vi "EMG_Control.vi"() -> ()   [LabVIEW 2015]
uses:
  <instrlib>/Dynamixel Motor/Public/Motor Operation/Low Level/Baud Setting.ctl
  <vilib>/Platform/TimedLoop/XDataNode/timing_clust.ctl
  <vilib>/Platform/TimedLoop/XDataNode/nitl_modes.ctl
  <vilib>/Platform/TimedLoop/XDataNode/wakeup.ctl
  <vilib>/platform/TimedLoop/XDataNode/XDataNode.xnode
  <instrlib>/Dynamixel Motor/Dynamixel Motor.lvlib
  <vilib>/Platform/TimedLoop/XDataNode/XDNodeRunTimeDep.lvlib
panel:
  out "Mover 4 motor info (degree)":T1(array[cluster]) {"Error Code (bits)" format="%b"}
  out "Hand motors info":T2(array[cluster])
  in  "Triceps max amplitude (V)":dbl
  in  "Biceps max amplitude (V)":dbl
  out "Mode":enum16{" M3", " M2", " M1"}(ring)
  in  "Positions":T3
  in  "Target IP Address":string="172.22.11.2"
  in  "VISA resource name":refnum<visa-resource-name>="COM9"
  in  "stop":bool
  out "Biceps EMG signal (V)":dbl[](graph)
  in  "Calibrate?":bool
  out "Biceps first threshold (V)":dbl
  out "Biceps second threshold (V)":dbl
  out "Triceps first threshold (V)":dbl
  out "Triceps second threshold (V)":dbl
  out "Triceps EMG signal (V)":dbl[](graph)
  out "Triceps hardly contracted?":bool
  out "Triceps contracted?":bool
  out "Biceps hardly contracted?":bool
  out "Biceps contracted?":bool
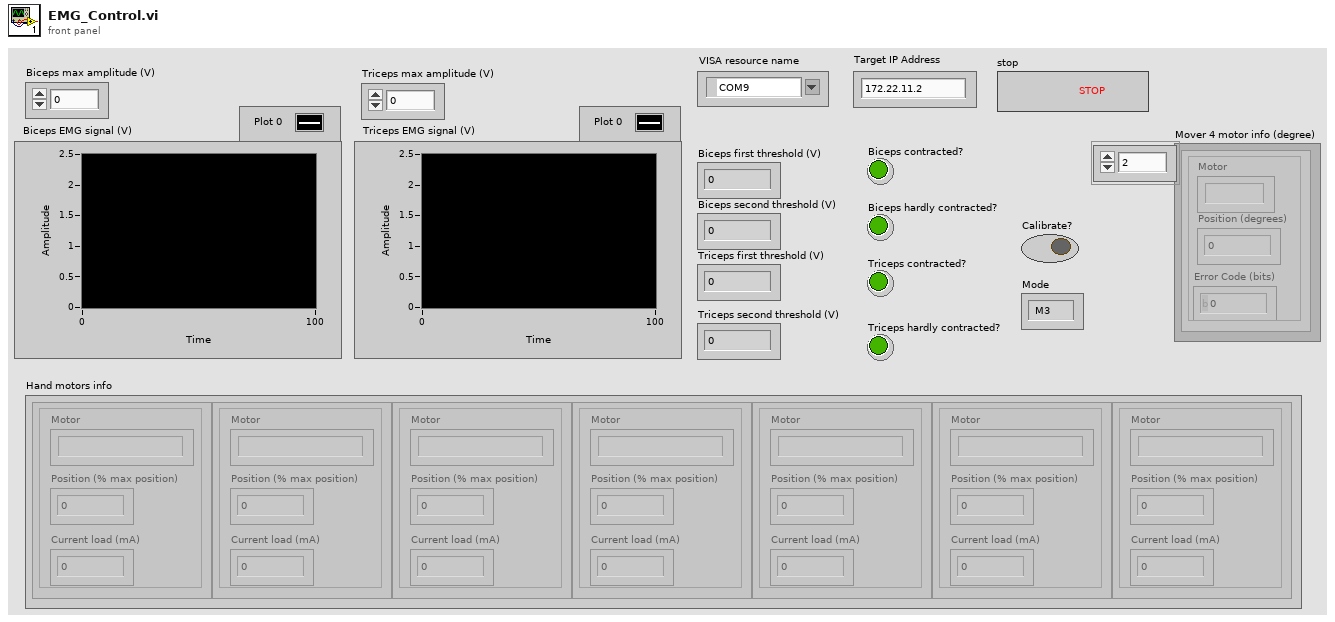
[diagram p1: front panel]
types:
  T1 = cluster{"Position (degrees)":i32, "Error Code (bits)":u8, "Motor":string}[]
  T2 = cluster{"Motor ":string, "Position (% max position)":dbl, "Current load (mA)":dbl}[]
  T3 = cluster{"ID":u16, "Position (bit)":u16, "Current load (mA)":u16}
  T4 = cluster{"Enable?":bool, "Reset?":bool, "EMG control":enum16{"Rest", "Biceps contracted", "Triceps contracted"}, "Motor speed":u8}
  T5 = cluster{"ID":u16, "Position (bit)":u16, "Current load (mA)":u16}[]
  T6 = cluster{"Read Access":enum8{"Allowed", "Required", "None"}, "Write Access":enum8{"Allowed", "Required", "None"}}
  T7 = cluster{"ID":u8, "Position":u16, "Error Code":u8}[]
  T8 = typedef "Dynamixel Motor.lvlib/Baud Setting.ctl" = u8
  T9 = typedef "XDNodeRunTimeDep.lvlib/timing_clust.ctl" = cluster{"Expected End [f-1]":u64, "Actual End [f-1]":u64, "Finished Late? [f-1]":bool, "Expected End [i-1]":u64, "Actual End [i-1]":u64, "Finished Late? [i-1]":bool, "Expected Start [i]":u64, "Actual Start [i]":u64, "Expected Start [f]":u64, "Actual Start [f]":u64, "Source Name":string, "Structure Name":string, "Period":i64, "Deadline":i64, "Offset":i64, "Start":i64, "Priority":i32, "Timeout":i32, "Mode":T10, "Wakeup Reason":T11, "Error":errorcluster, "Source Type":string, "Secondary Source Type":string, "Global End Time":u64, "Global Start Time":u64, "Frame Duration":u64, "Iteration Duration":u64, "Assigned CPU":i32, "I/O Scan Engine Mode":u32}
  T10 = typedef "XDNodeRunTimeDep.lvlib/nitl_modes.ctl" = enum32{"No Change", "Process missed periods, maintain original phase", "Discard missed periods, maintain original phase", "Process missed periods, ignore original phase", "Discard missed periods, ignore original phase"}
  T11 = typedef "XDNodeRunTimeDep.lvlib/wakeup.ctl" = enum32{"Normal", "Aborted", "Asynchronous wakeup", "Timing source error", "Timed loop error", "Timeout"}
  T12 = enum16{"Rest", "Triceps hardly contracted", "Triceps contracted", "Biceps hardly contracted", "Biceps contracted", "Change mode"}
  T13 = cluster{"Motor ":string, "Position (% Max position)":dbl, "Current load (mA)":dbl}[]
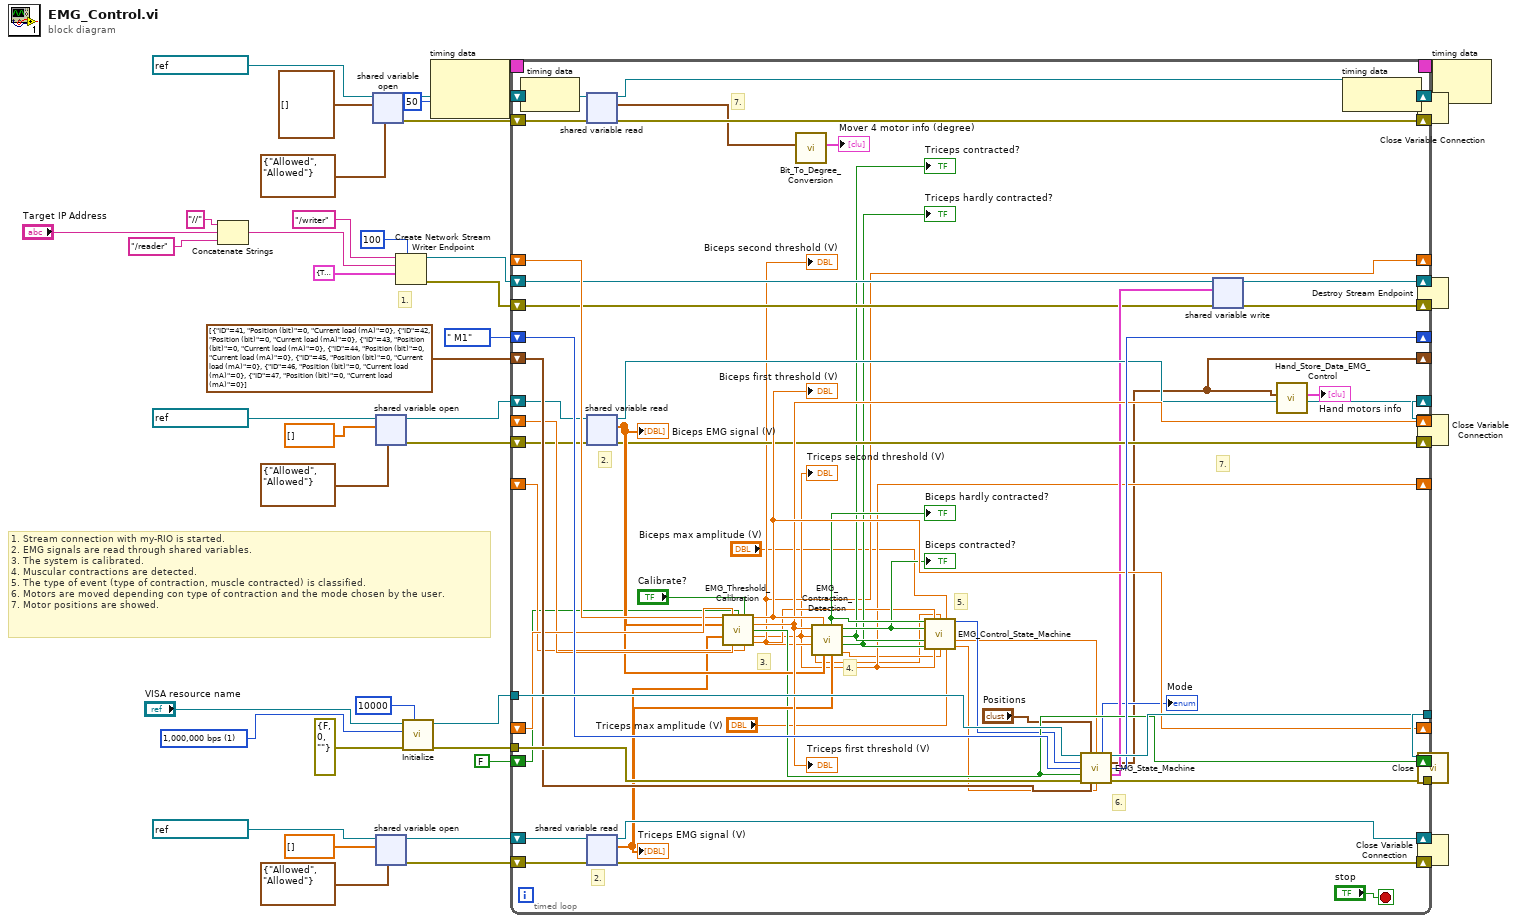
[diagram p0: block diagram]
diagram:
  w46 = T8 1 items=["1,000,000 bps"=1, "500,000 bps"=3, "400,000 bps"=4, "250,000 bps"=7, "200,000 bps"=9, "115200 bps"=16, "57600 bps"=34, "19200 bps"=103, "9600 bps"=207] ("Baud rate (57600 bps)")
  # "1."
  # "1. Stream connection with my-RIO is started.\n2. EMG signals are read through shared variables.\n3. The system is calibrated.\n4. Muscular contractions are detected.\n5. The type of event (type of contraction, muscle contracted) is classified.\n6. Motors are moved depending con type of contraction and the mode chosen by the user.\n7. Motor positions are showed."
  n1 = Concatenate Strings("//", "Target IP Address", "/reader") -> (w39:string)
  n2 = shared-variable-open(refnum<k21> "ni.var.psp://stratom-myrio/Shared_Variables/New position" ("shared variable refnum in"), T7 [] ("New position 2"), T6 {"Read Access"=enum."Allowed", "Write Access"=enum."Allowed"} ("access")) -> (w26:refnum<k21>, w24:errorcluster)  [unwired: 1 in]
  n3 = shared-variable-open(refnum<k21> "ni.var.psp://stratom-myrio/Shared_Variables/Biceps EMG signal" ("shared variable refnum in"), dbl[] [], T6 {"Read Access"=enum."Allowed", "Write Access"=enum."Allowed"} ("access")) -> (w18:refnum<k21>, w17:errorcluster)  [unwired: 1 in]
  n4 = shared-variable-open(refnum<k21> "ni.var.psp://stratom-myrio/Shared_Variables/Triceps EMG signal" ("shared variable refnum in"), dbl[] [], T6 {"Read Access"=enum."Allowed", "Write Access"=enum."Allowed"} ("access")) -> (w12:refnum<k21>, w11:errorcluster)  [unwired: 1 in]
  n5 = Create Network Stream Writer Endpoint(7:100 ("writer buffer size"), 9:T4 {"Enable?"=TRUE, "Reset?"=FALSE, "EMG control"=enum."Rest", "Motor speed"=0} ("data in"), 10:w39, 11:"/writer" ("reader name")) -> (0:w33:errorcluster, 3:w34:refnum<k21>)  [unwired: 3 in]
  n6 = call <instrlib>:"Initialize.vi"("Timeout (30 msec)"=u32 10000, "error in (no error)"=errorcluster {"status"=FALSE, "code"=0, "source"=""}, "Baud rate (57600 bps)"=w46, "VISA resource name"="VISA resource name") -> ("error out"=w41:errorcluster, "VISA resource name out"=w42:refnum<visa-resource-name>)  [unwired: 6 in]
  n7 = node-c288(i64 50 ("Period")) -> (w3:T9)  [unwired: 1 in]
  n8 = timed-loop {
    shift-right: [w85] -> _
    shift-left: _ -> [w89]
    shift-right: [w58] -> _
    shift-left: _ -> [w87]
    shift-right: [w84] -> _
    shift-left: _ -> [w88]
    shift-right: [w57] -> _
    shift-left: _ -> [w86]
    tunnel: w42 -> [w100]
    tunnel: w41 -> [w99]
    shift-right: [w66] -> w32
    shift-left: w34 -> [w67]
    shift-right: [w65] -> w31
    shift-left: w33 -> [w64]
    tunnel: [w97] -> w30
    tunnel: [w96] -> w29
    shift-right: [w95] -> _
    shift-left: enum16{" M3", " M2", " M1"}." M1" ("Mode Out") -> [w98]
    shift-right: [w50] -> _
    shift-left: T5 [{"ID"=41, "Position (bit)"=0, "Current load (mA)"=0}, {"ID"=42, "Position (bit)"=0, "Current load (mA)"=0}, {"ID"=43, "Position (bit)"=0, "Current load (mA)"=0}, {"ID"=44, "Position (bit)"=0, "Current load (mA)"=0}, {"ID"=45, "Position (bit)"=0, "Current load (mA)"=0}, {"ID"=46, "Position (bit)"=0, "Current load (mA)"=0}, {"ID"=47, "Position (bit)"=0, "Current load (mA)"=0}] ("New Hand Positions") -> [w94]
    shift-right: [w91] -> w23
    shift-left: w26 -> [w93]
    shift-right: [w90] -> w22
    shift-left: w24 -> [w92]
    shift-right: [w79] -> w10
    shift-left: w18 -> [w82]
    shift-right: [w78] -> w9
    shift-left: w17 -> [w81]
    shift-right: [w75] -> w8
    shift-left: w12 -> [w77]
    shift-right: [w74] -> w7
    shift-left: w11 -> [w76]
    shift-right: [w72] -> _
    shift-left: FALSE ("System calibrated?") -> [w71]
    timing: w3 -> [_]
    timing-out: [_] -> w2
    stop <- "stop" stop-if-true
    # "7."
    # "7."
    # "6."
    # "5."
    # "4."
    # "3."
    # "2."
    # "2."
    n9 = node-c288() -> ()  [unwired: 1 in, 1 out]
    n10 = shared-variable-read(w93, w92) -> (w91:refnum<k21>, w90:errorcluster, w48:T7)  [unwired: 1 out]
    n11 = shared-variable-read(w82, w81) -> (w79:refnum<k21>, w78:errorcluster, w80:dbl[])  [unwired: 1 out]
    "Biceps EMG signal (V)" <- w80
    n12 = shared-variable-read(w77, w76) -> (w75:refnum<k21>, w74:errorcluster, w73:dbl[])  [unwired: 1 out]
    "Triceps EMG signal (V)" <- w73
    n13 = call "EMG_Threshold_Calibration.vi"("Biceps harder contraction threshold in (V)"=w87, "Biceps contraction threshold in (V)"=w89, "System calibrated? (input)"=w71, "Calibrate?"="Calibrate?", "Biceps EMG signal (V)"=w80, "Triceps EMG signal (V)"=w73, "Triceps contraction threshold in (V)"=w88, "Triceps harderd contraction threshold in (V)"=w86) -> ("Biceps contraction threshold out (V)"=w85:dbl, "Triceps contraction threshold out (V)"=w84:dbl, "System calibrated?"=w72:bool, "Triceps harderd contraction threshold out (V)"=w57:dbl, "Biceps harder contraction threshold out (V)"=w58:dbl)  [unwired: 3 in]
    "Biceps first threshold (V)" <- w85
    "Biceps second threshold (V)" <- w58
    "Triceps first threshold (V)" <- w84
    "Triceps second threshold (V)" <- w57
    n14 = call "Bit_To_Degree_Conversion.vi"("Actual joints positions"=w48) -> ("Motor positions (degree)"=→"Mover 4 motor info (degree)":T1)  [unwired: 10 in]
    n15 = call "EMG_Contraction_Detection.vi"("Triceps EMG signal (V)"=w73, "Biceps EMG signal (V)"=w80, "Biceps contraction threshold (V)"=w85, "Biceps harder contraction threshold  (V)"=w58, "Triceps harderd contraction threshold  (V)"=w57, "Triceps contraction threshold  (V)"=w84) -> ("Triceps mean amplitude during contraction  (V)"=w56:dbl, "Triceps hardly contracted?"=w59:bool, "Triceps contracted?"=w60:bool, "Biceps contracted?"=w61:bool, "Biceps hardly contracted?"=w62:bool, "Biceps mean amplitude during contraction  (V)"=w55:dbl)
    "Triceps hardly contracted?" <- w59
    "Triceps contracted?" <- w60
    "Biceps hardly contracted?" <- w62
    "Biceps contracted?" <- w61
    n16 = call "EMG_Control_State_Machine.vi"("Biceps hardly contracted?"=w62, "Biceps second threshold (V)"=w58, "Biceps mean amplitude (V)"=w55, "Biceps max amplitude (V)"="Biceps max amplitude (V)", "Biceps contracted?"=w61, "Triceps contracted?"=w60, "Triceps hardly contracted?"=w59, "Triceps second threshold (V)"=w57, "Triceps mean amplitude (V)"=w56, "Triceps max amplitude (V)"="Triceps max amplitude (V)") -> ("EMG Control"=w63:T12, "EMG signal max amplitude (V)"=w54:dbl, "EMG signal mean amplitude (V)"=w53:dbl)  [unwired: 3 in]
    n17 = call "EMG_State_Machine.vi"("VISA Refnum in"=w100, "Positions"="Positions", "EMG signal max amplitude (V)"=w54, "EMG Control"=w63, "Mode in"=w98, "System calibrated?"=w72, "error in (no error)"=w99, "New Hand Positions in"=w94, "EMG signal mean amplitude (V)"=w53) -> ("Mode"=→"Mode":enum16{" M3", " M2", " M1"}, "VISA Refnum out"=w97:refnum<visa-resource-name>, "New Hand Positions out"=w50:T5, "Mode out"=w95:enum16{" M3", " M2", " M1"}, "Mover4 Data"=w70:T4, "error out"=w96:errorcluster)  [unwired: 1 in]
    n18 = shared-variable-write(w67, w64, w70) -> (w66:refnum<k21>, w65:errorcluster)  [unwired: 1 in, 1 out]
    n19 = call "Hand_Store_Data_EMG_Control.vi"("New Hand Positions"=w50) -> ("Hand motors info"=→"Hand motors info":T13)  [unwired: 10 in]
    n20 = node-c288() -> ()  [unwired: 1 in, 1 out]
  }
  n21 = Close Variable Connection(8:w22, 11:w23) -> ()  [unwired: 1 out]
  n22 = Destroy Stream Endpoint(8:w31, 11:w32) -> ()  [unwired: 1 out]
  n23 = Close Variable Connection(8:w9, 11:w10) -> ()  [unwired: 1 out]
  n24 = call <instrlib>:"Close.vi"("error in (no error)"=w29, "VISA resource name"=w30) -> ()  [unwired: 9 in, 1 out]
  n25 = Close Variable Connection(8:w7, 11:w8) -> ()  [unwired: 1 out]
  n26 = node-c288(w2) -> ()  [unwired: 1 out]
